vi "Write Pulse Configuration.vi"(8 "error in (no error)":errorcluster, 10 "Pulse Driver Configuration":T1={"Post-trigger delay"=0.01, "Post-trigger duration"=0.1, "Rate"=1000000.0, "Ranges"=[10.0], "Re-name channels"=[], "Active channels"="0:1", "External clock"=FALSE} {"Rate" format="%#_8pHz"; "Post-trigger duration" format="%#_6ps"; "Post-trigger delay" format="%#_6ps"; "Ranges" format="%#_6pV"}, 11 "Micron Optics Driver in":refnum<class "Micron Optics Driver.lvclass">) -> (0 "error out":errorcluster, 3 "Micron Optics Driver out":refnum<class "Micron Optics Driver.lvclass">)   [LabVIEW 2024, in "Micron Optics Driver.lvclass"]
uses:
  Micron Optics Driver.lvclass
  Pulse Driver/Pusle Driver Configuration.ctl
  Micron Optics Driver.lvclass/Micron Optics Driver.ctl
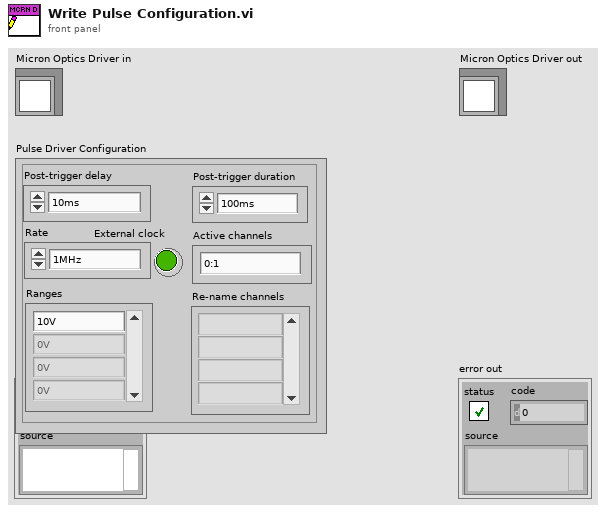
[diagram p1: front panel]
types:
  T1 = typedef "Pusle Driver Configuration.ctl" = cluster{"Post-trigger delay":dbl, "Post-trigger duration":dbl, "Rate":dbl, "Ranges":dbl[], "Re-name channels":string[], "Active channels":string, "External clock":bool}
  T2 = typedef "Micron optics didgitizer configuration.ctl" = cluster{"Post-trigger delay":dbl, "Post-trigger duration":dbl, "Rate":dbl, "Reference channel":i32, "Detection Setting IDs":u8[], "Stream and average":bool, "Address":string}
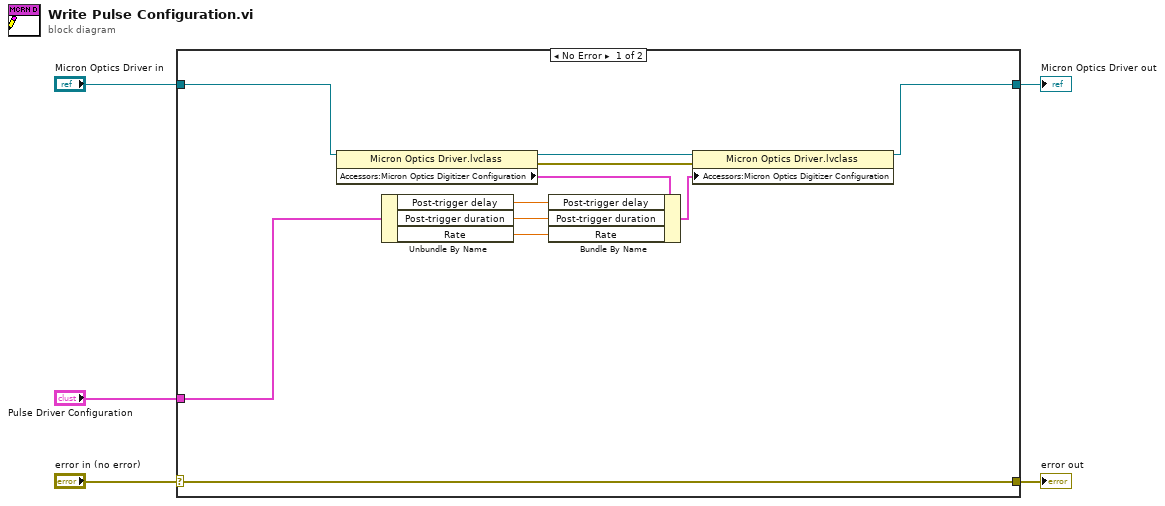
[diagram p0: block diagram]
diagram:
  n1 = case shown="No Error" "error in (no error)" {
    selector: "error in (no error)" -> [w16 w17]
    tunnel: [w16 w17] -> w4
    tunnel: [w8 w18] -> w2
    tunnel: "Micron Optics Driver in" -> [w7 w18]
    tunnel: "Pulse Driver Configuration" -> [w6 _]
    frame No Error {
      n2 = property class="Micron Optics Driver.lvclass"(reference=w7) -> (reference out=w9:refnum<class "Micron Optics Driver.lvclass">, error out=w15:errorcluster, "Accessors:Micron Optics Digitizer Configuration"=w10:T2)  [unwired: 1 in]
      n3 = Unbundle By Name(w6) -> ("Post-trigger delay"=w14:dbl, "Post-trigger duration"=w13:dbl, "Rate"=w12:dbl)
      n4 = Bundle By Name(cluster=w10, "Post-trigger delay"=w14, "Post-trigger duration"=w13, "Rate"=w12) -> (w11:T2)
      n5 = property class="Micron Optics Driver.lvclass"(reference=w9, error in=w15, "Accessors:Micron Optics Digitizer Configuration"=w11) -> (reference out=w8:refnum<class "Micron Optics Driver.lvclass">)  [unwired: 1 out]
    }
    frame Error {
    }
  }
  "error out" <- w4
  "Micron Optics Driver out" <- w2
